vi "FTW-CodeGen-GetTerms.vi"(0 "State In":T2 {"Width" format="%dpx"}, 5 "XRef":refnum<vi>) -> (4 "Terms":T1(array[cluster]))   [LabVIEW 2015, in "FTW-Dataflow-Burrow.xnode"]
uses:
  FTW-Dataflow-Burrow.xnode
  FTW-CodeGen-State.ctl
panel:
  # "Inputs"
  # "Outputs"
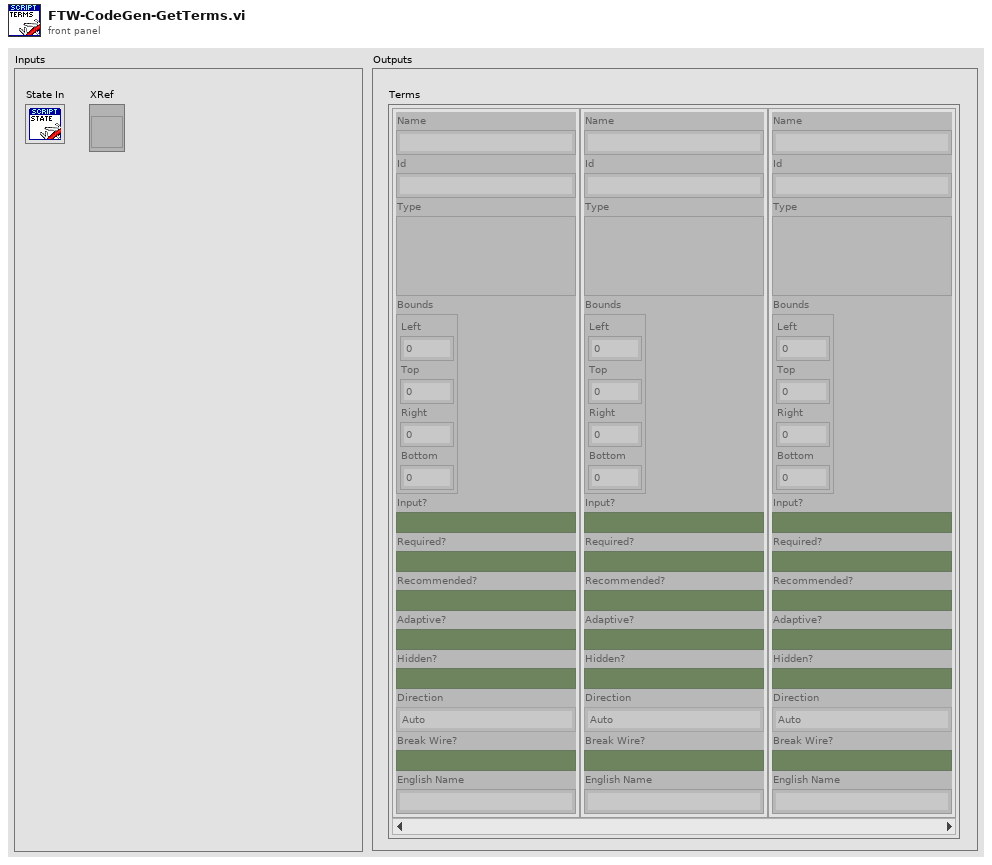
[diagram p1: front panel]
types:
  T1 = cluster{"Name":string, "Id":string, "Type":variant, "Bounds":cluster{"Left":i32, "Top":i32, "Right":i32, "Bottom":i32}, "Input?":bool, "Required?":bool, "Recommended?":bool, "Adaptive?":bool, "Hidden?":bool, "Direction":enum32{"Auto", "Up", "Down", "Left", "Right", "Center"}, "Break Wire?":bool, "English Name":string}[]
  T2 = typedef "FTW-Dataflow-Burrow.xnode/FTW-CodeGen-State.ctl" = cluster{"InputTerminals":cluster{"Wired?":bool, "ID":string, "DataName":string, "DataColor":u32, "Type":variant}[], "EnableTiming?":bool, "Width":i32}
  T3 = cluster{"Wired?":bool, "ID":string, "DataName":string, "DataColor":u32, "Type":variant}[]
  T4 = enum32{"Auto", "Up", "Down", "Left", "Right", "Center"}
  T5 = cluster{"Name":string, "ID":string, "Type":variant, "Bounds":cluster{"Left":i32, "Top":i32, "Right":i32, "Bottom":i32}, "Input?":bool, "Required?":bool, "Recommended?":bool, "Adaptive?":bool, "Hidden?":bool, "Direction":enum32{"Auto", "Up", "Down", "Left", "Right", "Center"}, "Break Wire?":bool, "English Name":string}
  T6 = cluster{"Name":string, "ID":string, "Type":variant, "Bounds":cluster{"Left":i32, "Top":i32, "Right":i32, "Bottom":i32}, "Input?":bool, "Required?":bool, "Recommended?":bool, "Adaptive?":bool, "Hidden?":bool, "Direction":enum32{"Auto", "Up", "Down", "Left", "Right", "Center"}, "Break Wire?":bool, "English Name":string}[]
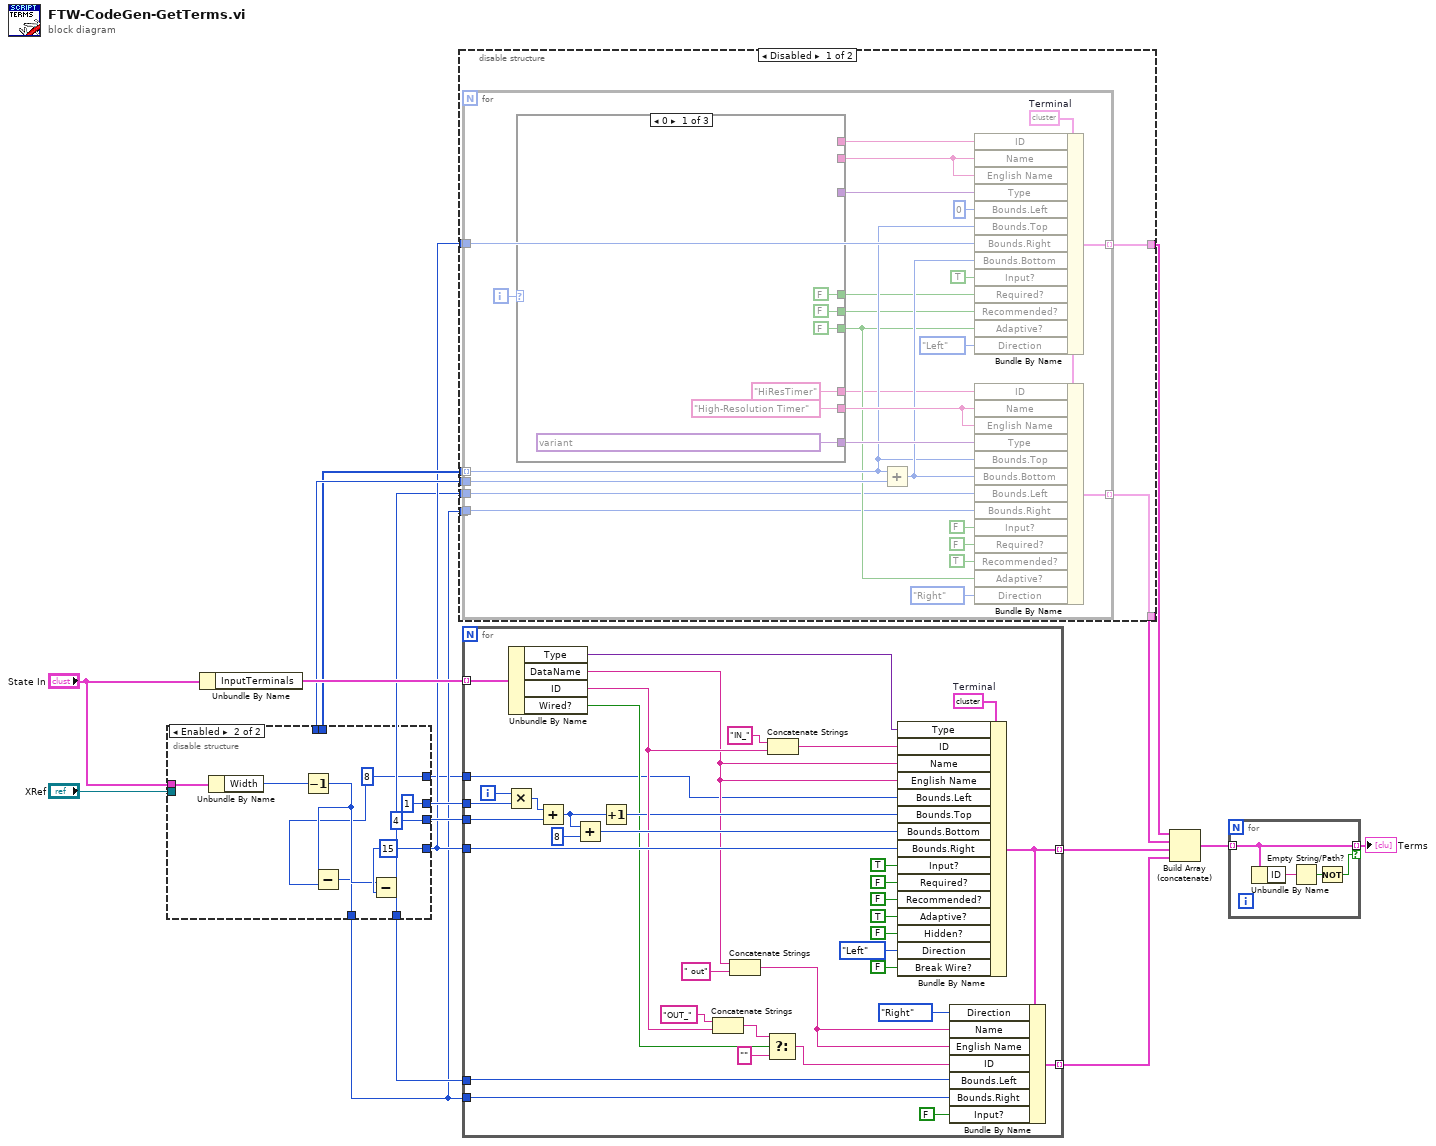
[diagram p0: block diagram]
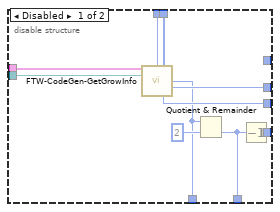
[diagram p2: hidden frame]
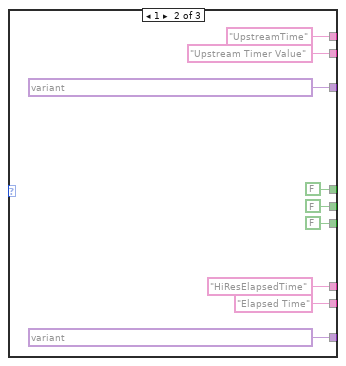
[diagram p3: hidden frame]
diagram:
  n1 = disable-structure shown="Enabled" {
    disable-tunnel: "State In" -> [w27 w34]
    disable-tunnel: "XRef" -> [w26 _]
    disable-tunnel: [w24 4 ("Total Top Banner Height")] -> w15
    disable-tunnel: [w23 1 ("Terminal Height")] -> w10
    disable-tunnel: [w22 _] -> w9
    disable-tunnel: [w21 _] -> w8
    disable-tunnel: [w20 w31] -> w5
    disable-tunnel: [w19 w32] -> w4
    disable-tunnel: [w18 w28] -> w3
    disable-tunnel: [_ w29] -> w1
    frame Disabled {
      n2 = call "FTW-CodeGen-GetGrowInfo.vi"("State In"=w27, "XRef"=w26) -> ("Timing Terminal Height"=w22:i32, "Timing Terminals"=w21:i32[], "Width"=w18:i32, "Terminal Height"=w23:i32, "Total Top Banner Height"=w24:i32)  [unwired: 5 in, 4 out]
      n3 = Quotient & Remainder(x=w18, y=2) -> (floor(x/y)=w19:i32)  [unwired: 1 out]
      n4 = Decrement(x=w19) -> (x-1=w20:i32)
    }
    frame Enabled {
      w31 = 15
      w29 = 8 ("Bounds.Left")
      n5 = Unbundle By Name(w34) -> ("Width"=w33:i32)
      n6 = Decrement(x=w33) -> (x-1=w30:i32)
      n7 = Subtract(x=w30, y=w29) -> (x-y=w28:i32)
      n8 = Subtract(x=w30, y=w31) -> (x-y=w32:i32)
    }
  }
  n9 = Unbundle By Name("State In") -> ("InputTerminals"=w14:T3)
  n10 = disable-structure shown="Disabled" {
    disable-tunnel: [w43 _] -> w11
    disable-tunnel: w9 -> [w42 _]
    disable-tunnel: w8 -> [w41 _]
    disable-tunnel: [w40 _] -> w7
    disable-tunnel: w5 -> [w39 _]
    disable-tunnel: w4 -> [w38 _]
    disable-tunnel: w3 -> [w37 _]
    frame Disabled {
      n11 = for {
        tunnel: [w68] -> w43 mode=indexing
        tunnel: w42 -> [w59]
        tunnel: w41 -> [w53] mode=indexing
        tunnel: [w64] -> w40 mode=indexing
        tunnel: w39 -> [w60]
        tunnel: w38 -> [w47]
        tunnel: w37 -> [w48]
        i -> [w51]
        w44 = T5 {"Name"="", "ID"="", "Type"=variant, "Bounds"={"Left"=0, "Top"=0, "Right"=0, "Bottom"=0}, "Input?"=FALSE, "Required?"=FALSE, "Recommended?"=FALSE, "Adaptive?"=FALSE, "Hidden?"=FALSE, "Direction"=enum."Auto", "Break Wire?"=FALSE, "English Name"=""}  # Terminal
        n12 = case shown="0" w51 {
          tunnel: [_ "Upstream Timer Value" ("Name") _] -> w69
          tunnel: [_ variant(dbl 0.0) ("variant") _] -> w67
          tunnel: ["High-Resolution Timer" ("Name") "Elapsed Time" ("Name") _] -> w61
          tunnel: [variant(dbl 0.0) ("variant") variant(dbl 0.0) ("variant") _] -> w62
          tunnel: [FALSE ("Required?") FALSE ("Required?") _] -> w50
          tunnel: [FALSE ("Recommended?") FALSE ("Recommended?") _] -> w49
          tunnel: [FALSE ("Adaptive?") FALSE ("Adaptive?") _] -> w52
          tunnel: [_ "UpstreamTime" ("ID") _] -> w45
          tunnel: ["HiResTimer" ("ID") "HiResElapsedTime" ("ID") _] -> w46
          frame 0 {
          }
          frame 1 {
          }
          frame Default {
          }
        }
        n13 = Add(x=w53, y=w59) -> (x+y=w58:i32)
        n14 = Bundle By Name(cluster=w44, "ID"=w45, "Name"=w69, "English Name"=w69, "Type"=w67, "Bounds.Left"=0, "Bounds.Top"=w53, "Bounds.Right"=w60, "Bounds.Bottom"=w58, "Input?"=TRUE, "Required?"=w50, "Recommended?"=w49, "Adaptive?"=w52, "Direction"=T4."Left") -> (w68:T5)
        n15 = Bundle By Name(cluster=w44, "ID"=w46, "Name"=w61, "English Name"=w61, "Type"=w62, "Bounds.Top"=w53, "Bounds.Bottom"=w58, "Bounds.Left"=w47, "Bounds.Right"=w48, "Input?"=FALSE, "Required?"=FALSE, "Recommended?"=TRUE, "Adaptive?"=w52, "Direction"=T4."Right") -> (w64:T5)
      }
    }
    frame Enabled {
    }
  }
  n16 = for {
    tunnel: w10 -> [w113]
    tunnel: w15 -> [w114]
    tunnel: w5 -> [w110]
    tunnel: w3 -> [w111]
    tunnel: w4 -> [w112]
    tunnel: w14 -> [w107] mode=indexing
    tunnel: [w104] -> w13 mode=indexing
    tunnel: [w103] -> w12 mode=indexing
    tunnel: w1 -> [w86]
    i -> [w106]
    w97 = T5 {"Name"="", "ID"="", "Type"=variant, "Bounds"={"Left"=0, "Top"=0, "Right"=0, "Bottom"=0}, "Input?"=FALSE, "Required?"=FALSE, "Recommended?"=FALSE, "Adaptive?"=FALSE, "Hidden?"=FALSE, "Direction"=enum."Auto", "Break Wire?"=FALSE, "English Name"=""}  # Terminal
    n17 = Multiply(x=w106, y=w113) -> (x*y=w115:i32)
    n18 = Unbundle By Name(w107) -> ("Type"=w91:variant, "DataName"=w90:string, "ID"=w98:string, "Wired?"=w89:bool)
    n19 = Add(x=w115, y=w114) -> (x+y=w109:i32)
    n20 = Add(x=w109, y=8) -> (x+y=w108:i32)
    n21 = Increment(x=w109) -> (x+1=w92:i32)
    n22 = Concatenate Strings("OUT_" ("format string"), w98) -> (w95:string)
    n23 = Concatenate Strings(w90, " out" ("string")) -> (w93:string)
    n24 = Select(t=w95, s=w89, f="") -> (s? t:f=w87:string)
    n25 = Concatenate Strings("IN_" ("format string"), w98) -> (w88:string)
    n26 = Bundle By Name(cluster=w97, "Type"=w91, "ID"=w88, "Name"=w90, "English Name"=w90, "Bounds.Left"=w86, "Bounds.Top"=w92, "Bounds.Bottom"=w108, "Bounds.Right"=w110, "Input?"=TRUE, "Required?"=FALSE, "Recommended?"=FALSE, "Adaptive?"=TRUE, "Hidden?"=FALSE, "Direction"=T4."Left", "Break Wire?"=FALSE) -> (w104:T5)
    n27 = Bundle By Name(cluster=w104, "Direction"=T4."Right", "Name"=w93, "English Name"=w93, "ID"=w87, "Bounds.Left"=w112, "Bounds.Right"=w111, "Input?"=FALSE) -> (w103:T5)
  }
  n28 = Build Array (concatenate)(w11, w7, w13, w12) -> (w2:T6)
  n29 = for {
    tunnel: w2 -> [w125] mode=indexing
    tunnel: [w125] -> w6 mode=indexing if=w122
    n30 = Unbundle By Name(w125) -> ("ID"=w123:string)
    n31 = Empty String/Path?(string/path=w123) -> (empty?=w124:bool)
    n32 = Not(x=w124) -> (.not. x?=w122:bool)
  }
  "Terms" <- w6
